vi "Acc_Y.vi"(1 "y_ini":dbl) -> (0 "y_Acc":dbl)   [LabVIEW 2010]
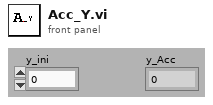
[diagram p1: front panel]
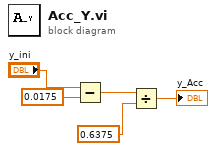
[diagram p0: block diagram]
diagram:
  n1 = Subtract(x="y_ini", y=0.0175) -> (x-y=w3:dbl)
  n2 = Divide(x=w3, y=0.6375) -> (x/y=→"y_Acc":dbl)
